vi "Automatic Shooter Sequence.vi"() -> ()   [LabVIEW 2012]
uses:
  Robot Global Data.vi
panel:
  out "Loop Time 2":u32(graph)
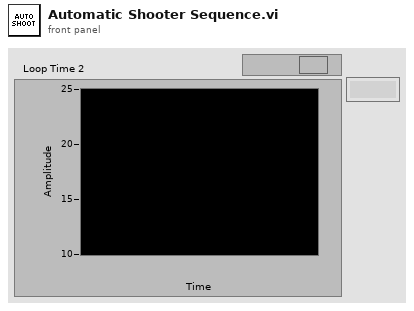
[diagram p1: front panel]
types:
  T1 = enum16{"Shooter Off", "Shooter On", "Extend Plunger"}
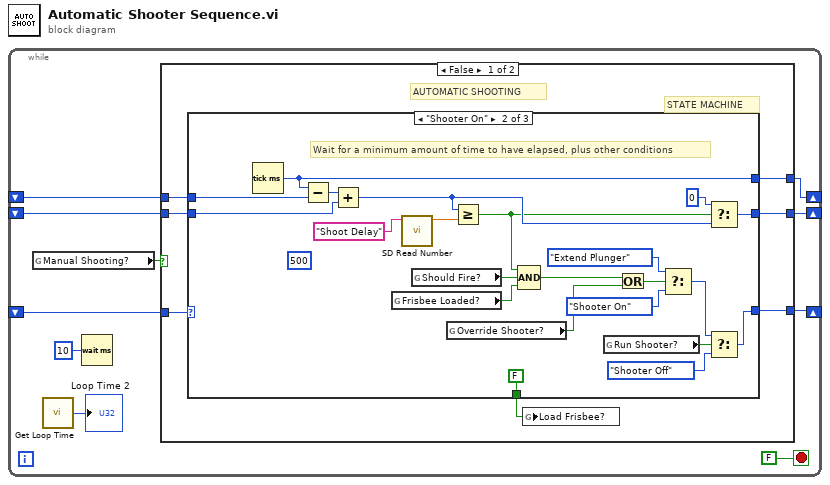
[diagram p0: block diagram]
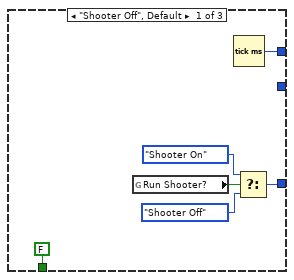
[diagram p2: hidden frame]
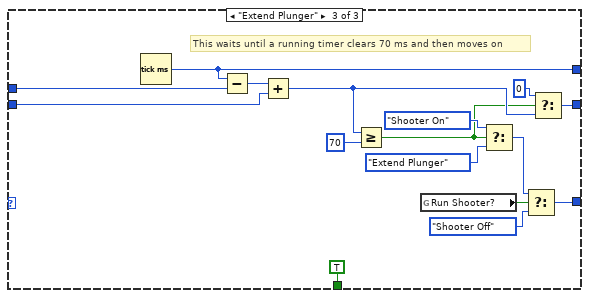
[diagram p3: hidden frame]
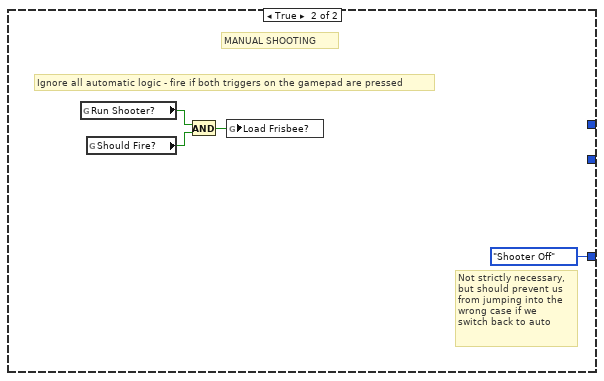
[diagram p4: hidden frame]
diagram:
  n1 = while {
    shift-right: [w1] -> _
    shift-left: _ -> [w9]
    shift-right: [w5] -> _
    shift-left: _ -> [w6]
    shift-right: [w3] -> _
    shift-left: _ -> [w4]
    stop <- FALSE stop-if-true
    n2 = global read "Robot Global Data.vi" "Manual Shooting?"() -> (w7:bool)
    n3 = call "Get Loop Time.vi"() -> ("Loop Time"=→"Loop Time 2":u32)  [unwired: 1 in]
    n4 = Wait (ms)(milliseconds to wait=u32 10) -> ()  [unwired: 1 out]
    n5 = case shown="False" w7 {
      tunnel: w9 -> [w17 _]
      tunnel: w6 -> [w16 _]
      tunnel: [w15 _] -> w5
      tunnel: w4 -> [w14 _]
      tunnel: [w13 _] -> w3
      tunnel: [w11 T1."Shooter Off" ("State")] -> w1
      frame False {
        # "STATE MACHINE"
        # "AUTOMATIC SHOOTING"
        n6 = case shown="\"Shooter On\"" w17 {
          tunnel: [w23 w36 w51] -> w11
          tunnel: w16 -> [_ w31 w58]
          tunnel: [w18 w32 w57] -> w15
          tunnel: w14 -> [_ w30 w56]
          tunnel: [_ w26 w49] -> w13
          tunnel: [FALSE ("Plunger Extended?") FALSE ("Plunger Extended?") TRUE ("Plunger Extended?")] -> w12
          frame "Shooter Off", Default {
            n7 = global read "Robot Global Data.vi" "Run Shooter?"() -> (w22:bool)
            n8 = Tick Count (ms)() -> (millisecond timer value=w18:u32)
            n9 = Select(t=T1."Shooter On" ("State"), s=w22, f=T1."Shooter Off" ("State")) -> (s? t:f=w23:T1)
          }
          frame "Shooter On" {
            (unwired) u32 500 ("y")
            # "Wait for a minimum amount of time to have elapsed, plus other conditions"
            n10 = Tick Count (ms)() -> (millisecond timer value=w32:u32)
            n11 = Subtract(x=w32, y=w31) -> (x-y=w33:u32)
            n12 = Add(x=w33, y=w30) -> (x+y=w28:u32)
            n13 = global read "Robot Global Data.vi" "Frisbee Loaded?"() -> (w40:bool)
            n14 = call <vilib>:"SD Read Number.vi"("Name"="Shoot Delay") -> ("Numeric"=w25:dbl)  [unwired: 8 in, 2 out]
            n15 = global read "Robot Global Data.vi" "Should Fire?"() -> (w34:bool)
            n16 = global read "Robot Global Data.vi" "Override Shooter?"() -> (w42:bool)
            n17 = Greater Or Equal?(x=w28, y=w25) -> (x >= y?=w27:bool)
            n18 = Compound Arithmetic op=AND(w27, w34, w40) -> (w41:bool)
            n19 = global read "Robot Global Data.vi" "Run Shooter?"() -> (w45:bool)
            n20 = Or(x=w41, y=w42) -> (x .or. y?=w44:bool)
            n21 = Select(t=T1."Extend Plunger" ("State"), s=w44, f=T1."Shooter On" ("State")) -> (s? t:f=w43:T1)
            n22 = Select(t=u32 0, s=w27, f=w28) -> (s? t:f=w26:u32)
            n23 = Select(t=w43, s=w45, f=T1."Shooter Off" ("State")) -> (s? t:f=w36:T1)
          }
          frame "Extend Plunger" {
            # "This waits until a running timer clears 70 ms and then moves on"
            n24 = Tick Count (ms)() -> (millisecond timer value=w57:u32)
            n25 = Subtract(x=w57, y=w58) -> (x-y=w59:u32)
            n26 = Add(x=w59, y=w56) -> (x+y=w48:u32)
            n27 = Greater Or Equal?(x=w48, y=u32 70) -> (x >= y?=w47:bool)
            n28 = global read "Robot Global Data.vi" "Run Shooter?"() -> (w61:bool)
            n29 = Select(t=T1."Shooter On" ("State"), s=w47, f=T1."Extend Plunger" ("State")) -> (s? t:f=w60:T1)
            n30 = Select(t=w60, s=w61, f=T1."Shooter Off" ("State")) -> (s? t:f=w51:T1)
            n31 = Select(t=u32 0, s=w47, f=w48) -> (s? t:f=w49:u32)
          }
        }
        n32 = global write "Robot Global Data.vi" "Load Frisbee?"(w12) -> ()
      }
      frame True {
        # "MANUAL SHOOTING"
        # "Ignore all automatic logic - fire if both triggers on the gamepad are pressed"
        # "Not strictly necessary,\nbut should prevent us\nfrom jumping into the\nwrong case if we\nswitch back to auto"
        n33 = global read "Robot Global Data.vi" "Run Shooter?"() -> (w65:bool)
        n34 = global read "Robot Global Data.vi" "Should Fire?"() -> (w63:bool)
        n35 = And(x=w65, y=w63) -> (x .and. y?=w64:bool)
        n36 = global write "Robot Global Data.vi" "Load Frisbee?"(w64) -> ()
      }
    }
  }
